vi "User message window-positioning management FG.vi"(9 "Function (\"Manage\")":T2, 11 "Default Window position (in)":T1) -> (2 "Default Window position":T1, 3 "New window position to set":T1)   [LabVIEW 2013]
uses:
  <vilib>/Utility/miscctls.llb/LVRectTypeDef.ctl
  Typedefs/Window position FG states.ctl
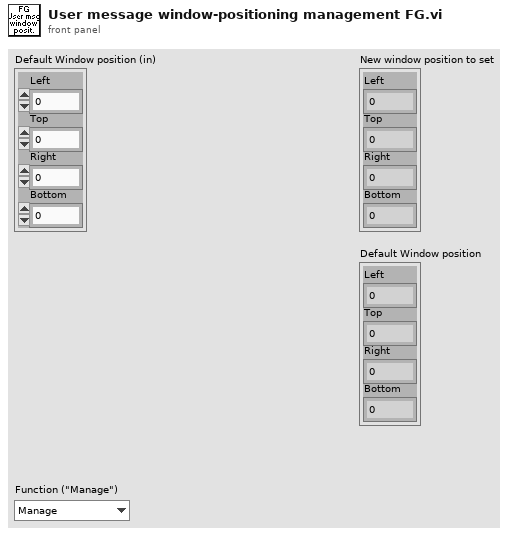
[diagram p1: front panel]
types:
  T1 = typedef "LVRectTypeDef.ctl" = cluster{"Left":i16, "Top":i16, "Right":i16, "Bottom":i16}
  T2 = typedef "Window position FG states.ctl" = enum16{"Manage", "Query", "Write"}
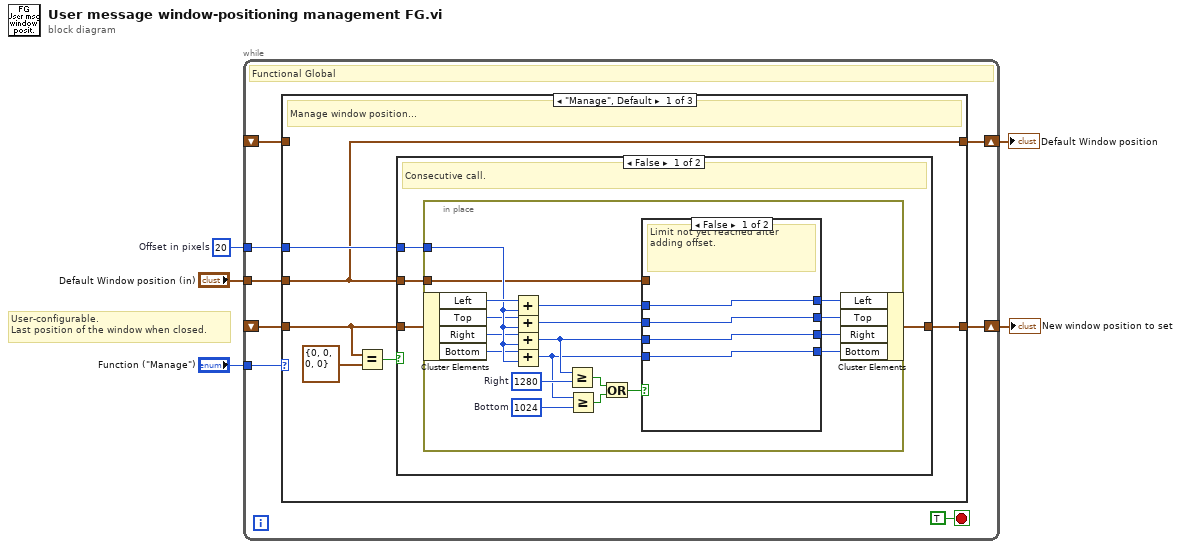
[diagram p0: block diagram]
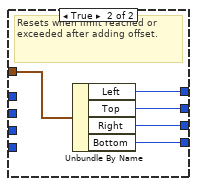
[diagram p2: hidden frame]
diagram:
  w2 = i16 20  # Offset in pixels
  # "User-configurable.\nLast position of the window when closed."
  n1 = while {
    shift-right: [w12] -> w5
    shift-left: _ -> [w9]
    tunnel: "Default Window position (in)" -> [w11]
    tunnel: w2 -> [w10]
    tunnel: "Function (\"Manage\")" -> [w8]
    shift-right: [w7] -> w1
    shift-left: _ -> [w6]
    stop <- TRUE stop-if-true
    # "Functional Global"
    n2 = case shown="\"Manage\", Default" w8 {
      tunnel: [w19 w54 w55] -> w12
      tunnel: w11 -> [w14 _ w55]
      tunnel: w10 -> [w18 _ _]
      tunnel: w9 -> [w16 w54 _]
      tunnel: [w14 w53 w56] -> w7
      tunnel: w6 -> [_ w53 w56]
      frame "Manage", Default {
        # "Manage window position..."
        n3 = Equal?(x=w16, y=T1 {"Left"=0, "Top"=0, "Right"=0, "Bottom"=0} ("Actual Window position (in)")) -> (x = y?=w17:bool)
        n4 = case shown="False" w17 {
          tunnel: [w22 w52] -> w19
          tunnel: w14 -> [w21 w52]
          tunnel: w18 -> [w23 _]
          tunnel: w16 -> [w20 _]
          frame False {
            # "Consecutive call."
            n5 = in-place {
              in-place-border: w23 -> [w41]
              in-place-border: w21 -> [w28]
              w34 = i16 1024  # Bottom
              w35 = i16 1280  # Right
              n6 = in-place-cluster #1(w20) -> ("Left"=w42:i16, "Top"=w40:i16, "Right"=w39:i16, "Bottom"=w38:i16)
              n7 = Add(x=w42, y=w41) -> (x+y=w32:i16)
              n8 = Add(x=w40, y=w41) -> (x+y=w31:i16)
              n9 = Add(x=w39, y=w41) -> (x+y=w30:i16)
              n10 = Add(x=w38, y=w41) -> (x+y=w29:i16)
              n11 = Greater Or Equal?(x=w30, y=w35) -> (x >= y?=w37:bool)
              n12 = Greater Or Equal?(x=w29, y=w34) -> (x >= y?=w36:bool)
              n13 = Or(x=w37, y=w36) -> (x .or. y?=w33:bool)
              n14 = case shown="False" w33 {
                tunnel: w32 -> [w46 _]
                tunnel: [w46 w50] -> w27
                tunnel: w31 -> [w45 _]
                tunnel: [w45 w49] -> w26
                tunnel: [w44 w48] -> w25
                tunnel: [w43 w47] -> w24
                tunnel: w30 -> [w44 _]
                tunnel: w29 -> [w43 _]
                tunnel: w28 -> [_ w51]
                frame False {
                  # "Limit not yet reached after adding offset."
                }
                frame True {
                  # "Resets when limit reached or exceeded after adding offset."
                  n15 = Unbundle By Name(w51) -> ("Left"=w50:i16, "Top"=w49:i16, "Right"=w48:i16, "Bottom"=w47:i16)
                }
              }
              n16 = in-place-cluster #1("Left"=w27, "Top"=w26, "Right"=w25, "Bottom"=w24) -> (w22:T1)
            }
          }
          frame True {
            # "First call / FG is empty."
          }
        }
      }
      frame "Query" {
        # "Query"
      }
      frame "Write" {
        # "Query"
      }
    }
  }
  "New window position to set" <- w5
  "Default Window position" <- w1
